vi "Process Repository.vi"(0 "Process In":refnum<class "Process.lvclass">, 5 "Action(ReadRepository)":T4(ring), 11 "Error In":errorcluster) -> (4 "Process Out":refnum<class "Process.lvclass">, 6 "ToProcessQueue":T2, 8 "ProcessAlreadyStarted":bool, 12 "ProcessViRef":refnum<vi>, 13 "ProcessSyncQueue":T3, 14 "FromProcessQueue":T1, 15 "Error Out":errorcluster)   [LabVIEW 2023, in "Process.lvclass"]
doc: "Governs the class object repository, in particular:\n- creates queues for new Process object, \n- allows impelement singleton pattern, \n- handles accesing to the process object queues,\n- menages liftime of queue storing process queues."
uses:
  Process.lvclass
  Interfaces/ICanCommunicate/ProcessSyncQueue.ctl
  Interfaces/ICanCommunicate/Message.ctl
  Interfaces/ICanCommunicate/ToProcessQueue.ctl
  Interfaces/ICanCommunicate/FromProcessQueue.ctl
  Interfaces/ICanCommunicate/Process Refs.ctl
  Process.lvclass/Process.ctl
  Process.vi
  Interfaces/ICanCommunicate/ICanCommunicate.lvclass
panel:
  # "Use this indicator for sending messages to the Process VI"
  # "These indicators are used by the process VIs"
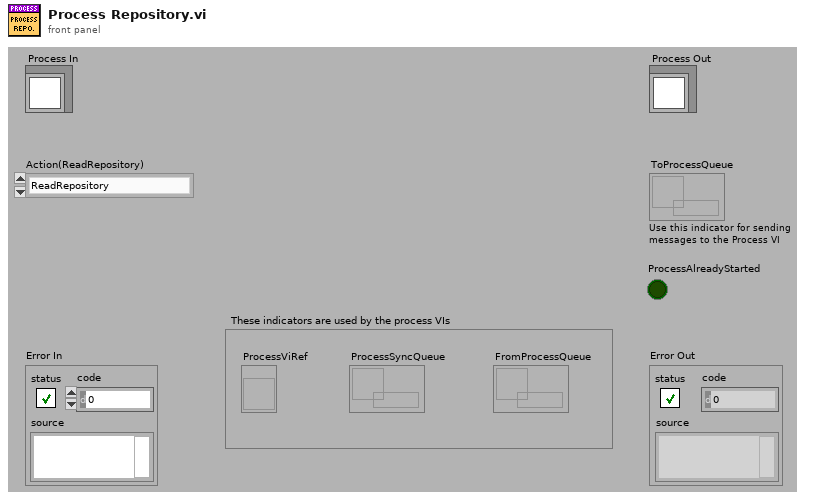
[diagram p1: front panel]
types:
  T1 = typedef "ICanCommunicate.lvclass/FromProcessQueue.ctl" = refnum<queue>
  T2 = typedef "ICanCommunicate.lvclass/ToProcessQueue.ctl" = refnum<queue>
  T3 = typedef "ICanCommunicate.lvclass/ProcessSyncQueue.ctl" = refnum<queue>
  T4 = enum16{"ReadRepository", "CreateNew", "CreateOrLookUpExisting", "ReadRepositoryAndDestroy"}
  T5 = typedef "ICanCommunicate.lvclass/Process Refs.ctl" = cluster{"ToProcessQueue":T2, "FromProcessQueue":T1, "ProcessSyncQueue":T3, "ProcessViRef":refnum<vi>}
  T6 = typedef "ICanCommunicate.lvclass/Message.ctl" = cluster{"Sender Name":string, "Recipent Name":string, "Command":string, "Data":variant, "Signature":string}
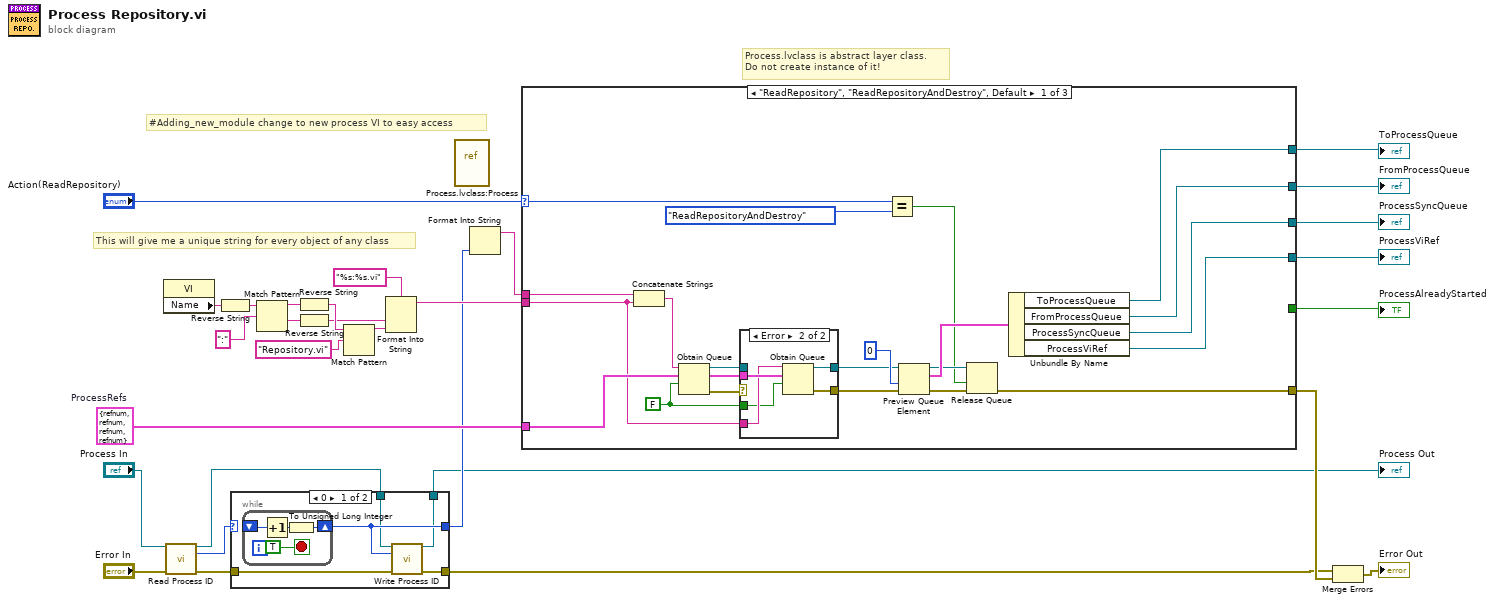
[diagram p0: block diagram]
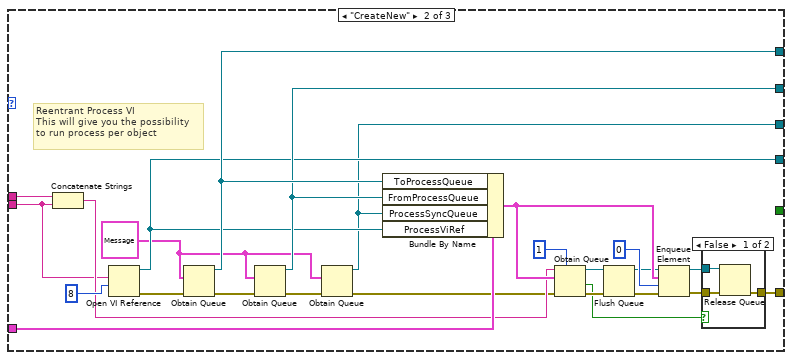
[diagram p4: hidden frame]
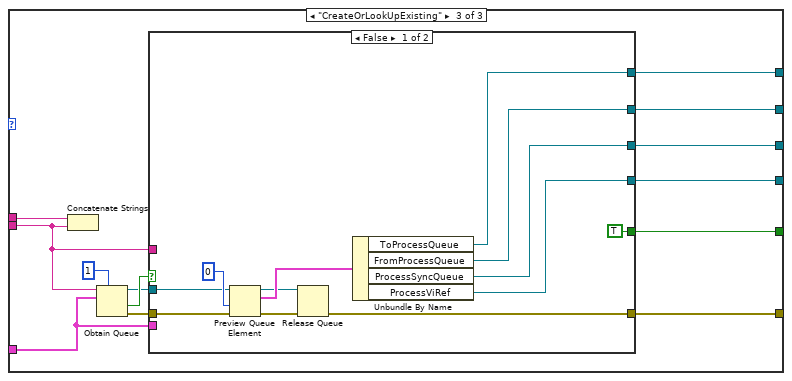
[diagram p6: hidden frame]
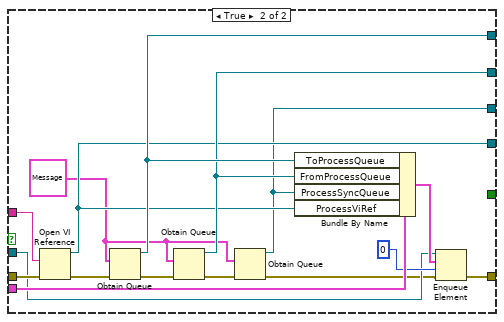
[diagram p7: hidden frame]
diagram:
  w24 = T5 {"ToProcessQueue"=refnum, "FromProcessQueue"=refnum, "ProcessSyncQueue"=refnum, "ProcessViRef"=refnum}  # ProcessRefs
  # "Process.lvclass is abstract layer class. \nDo not create instance of it!"
  # "#Adding_new_module change to new process VI to easy access"
  # "This will give me a unique string for every object of any class"
  n1 = property class="VI"() -> ("Name"=w13:string)  [unwired: 2 in, 2 out]
  n2 = call "Read Process ID.vi"("Process In"="Process In", "Error In"="Error In") -> ("Process Out"=w4:refnum<class "Process.lvclass">, "Process ID"=w2:u32, "Error Out"=w6:errorcluster)  [unwired: 11 in]
  n3 = Reverse String(1:w13) -> (0:w14:string)
  n4 = case shown="0" w2 {
    selector: w2 -> [_ w40]
    tunnel: [w34 w40] -> w7
    tunnel: w4 -> [w33 w41]
    tunnel: [w32 w41] -> w3
    tunnel: w6 -> [w31 w39]
    tunnel: [w30 w39] -> w8
    frame 0 {
      n5 = while {
        shift-right: [w35] -> w34
        shift-left: _ -> [w37]
        stop <- TRUE stop-if-true
        n6 = Increment(x=w37) -> (x+1=w36:u32)
        n7 = To Unsigned Long Integer(number=w36) -> (unsigned 32bit integer=w35:u32)
      }
      n8 = call "Write Process ID.vi"("Process In"=w33, "Process ID"=w34, "Error In"=w31) -> ("Process Out"=w32:refnum<class "Process.lvclass">, "Error Out"=w30:errorcluster)  [unwired: 11 in]
    }
    frame Default {
    }
  }
  "Process Out" <- w3
  n9 = Match Pattern(string=w14, regular expression=":") -> (before substring=w18:string, after substring=w15:string)  [unwired: 1 in, 2 out]
  n10 = Reverse String(1:w18) -> (0:w19:string)
  n11 = Reverse String(1:w15) -> (0:w17:string)
  n12 = Match Pattern(string=w19, regular expression="Repository.vi") -> (before substring=w21:string)  [unwired: 1 in, 3 out]
  n13 = Format Into String(format string="%s:%s.vi", w17, w21) -> (resulting string=w11:string)  [unwired: 2 in, 1 out]
  n14 = vi-ref "Process.lvclass:Process.vi"() -> ()  [unwired: 1 out]
  n15 = Format Into String(w7) -> (resulting string=w9:string)  [unwired: 3 in, 1 out]
  n16 = case shown="\"ReadRepository\", \"ReadRepositoryAndDestroy\", Default" "Action(ReadRepository)" {
    selector: "Action(ReadRepository)" -> [w43 _ _]
    tunnel: [w57 w78 w109] -> w28
    tunnel: [w59 w94 w111] -> w26
    tunnel: [w58 w93 w110] -> w27
    tunnel: [w60 w92 w108] -> w25
    tunnel: w24 -> [w52 w84 w104]
    tunnel: w9 -> [w50 w83 w100]
    tunnel: [w45 w72 w107] -> w22
    tunnel: w11 -> [w49 w81 w99]
    tunnel: [_ _ w102] -> w10
    frame "ReadRepository", "ReadRepositoryAndDestroy", Default {
      w51 = FALSE ("create if not found? (T)")
      n17 = Concatenate Strings(w50, w49) -> (w48:string)
      n18 = Obtain Queue(name (unnamed)=w48, element data type=w52, create if not found? (T)=w51) -> (queue out=w54:refnum<queue>, error out=w56:errorcluster)  [unwired: 2 in, 1 out]
      n19 = case shown="Error" w56 {
        selector: w56 -> [w64 _]
        tunnel: [w64 w66] -> w55
        tunnel: w54 -> [w63 _]
        tunnel: [w63 w67] -> w53
        tunnel: w52 -> [_ w69]
        tunnel: w49 -> [_ w68]
        tunnel: w51 -> [_ w65]
        frame No Error {
        }
        frame Error {
          n20 = Obtain Queue(name (unnamed)=w68, element data type=w69, create if not found? (T)=w65) -> (queue out=w67:refnum<queue>, error out=w66:errorcluster)  [unwired: 2 in, 1 out]
        }
      }
      n21 = Equal?(x=w43, y=T4."ReadRepositoryAndDestroy") -> (x = y?=w42:bool)
      n22 = Preview Queue Element(queue=w53, timeout in ms (-1)=0, error in (no error)=w55) -> (queue out=w47:refnum<queue>, element=w61:T5, error out=w46:errorcluster)  [unwired: 1 out]
      n23 = Release Queue(queue=w47, force destroy? (F)=w42, error in (no error)=w46) -> (error out=w45:errorcluster)  [unwired: 2 out]
      n24 = Unbundle By Name(w61) -> ("ToProcessQueue"=w59:T2, "FromProcessQueue"=w58:T1, "ProcessSyncQueue"=w57:T3, "ProcessViRef"=w60:refnum<vi>)
    }
    frame "CreateNew" {
      w70 = T6 {"Sender Name"="", "Recipent Name"="", "Command"="", "Data"=variant, "Signature"=""} ("Message")
      # "Reentrant Process VI\nThis will give you the possibility\nto run process per object"
      n25 = Concatenate Strings(w83, w81) -> (w82:string)
      n26 = Open VI Reference(vi path=w81, options=8 ("Reentrant Process VI\nThis will give you the possibility\nto run process per object")) -> (vi reference=w92:refnum<vi>, error out=w90:errorcluster)  [unwired: 4 in]
      n27 = Obtain Queue(element data type=w70, error in (no error)=w90) -> (queue out=w94:refnum<queue>, error out=w91:errorcluster)  [unwired: 3 in, 1 out]
      n28 = Obtain Queue(element data type=w70, error in (no error)=w91) -> (queue out=w93:refnum<queue>, error out=w80:errorcluster)  [unwired: 3 in, 1 out]
      n29 = Obtain Queue(element data type=w70, error in (no error)=w80) -> (queue out=w78:refnum<queue>, error out=w79:errorcluster)  [unwired: 3 in, 1 out]
      n30 = Bundle By Name(cluster=w84, "ToProcessQueue"=w94, "FromProcessQueue"=w93, "ProcessSyncQueue"=w78, "ProcessViRef"=w92) -> (w87:T5)
      n31 = Obtain Queue(max queue size (-1, unlimited)=1, name (unnamed)=w82, element data type=w87, error in (no error)=w79) -> (queue out=w88:refnum<queue>, created new?=w71:bool, error out=w76:errorcluster)  [unwired: 1 in]
      n32 = Flush Queue(queue=w88, error in (no error)=w76) -> (queue out=w77:refnum<queue>, error out=w75:errorcluster)  [unwired: 1 out]
      n33 = Enqueue Element(queue=w77, element=w87, timeout in ms (-1)=0, error in (no error)=w75) -> (queue out=w74:refnum<queue>, error out=w73:errorcluster)  [unwired: 1 out]
      n34 = case shown="False" w71 {
        tunnel: w73 -> [w97 w98]
        tunnel: w74 -> [w96 _]
        tunnel: [w95 w98] -> w72
        frame False {
          n35 = Release Queue(queue=w96, error in (no error)=w97) -> (error out=w95:errorcluster)  [unwired: 1 in, 2 out]
        }
        frame True {
        }
      }
    }
    frame "CreateOrLookUpExisting" {
      n36 = Concatenate Strings(w100, w99) -> ()  [unwired: 1 out]
      n37 = Obtain Queue(max queue size (-1, unlimited)=1, name (unnamed)=w99, element data type=w104) -> (queue out=w105:refnum<queue>, created new?=w106:bool, error out=w103:errorcluster)  [unwired: 2 in]
      n38 = case shown="False" w106 {
        tunnel: [w123 w139] -> w111
        tunnel: [w122 w138] -> w110
        tunnel: [w121 w125] -> w109
        tunnel: [w120 w137] -> w108
        tunnel: [w112 w136] -> w107
        tunnel: w104 -> [_ w135]
        tunnel: w103 -> [w117 w130]
        tunnel: w99 -> [_ w129]
        tunnel: w105 -> [w118 w128]
        tunnel: [TRUE _] -> w102
        frame False {
          n39 = Preview Queue Element(queue=w118, timeout in ms (-1)=0, error in (no error)=w117) -> (queue out=w114:refnum<queue>, element=w116:T5, error out=w113:errorcluster)  [unwired: 1 out]
          n40 = Release Queue(queue=w114, error in (no error)=w113) -> (error out=w112:errorcluster)  [unwired: 1 in, 2 out]
          n41 = Unbundle By Name(w116) -> ("ToProcessQueue"=w123:T2, "FromProcessQueue"=w122:T1, "ProcessSyncQueue"=w121:T3, "ProcessViRef"=w120:refnum<vi>)
        }
        frame True {
          w124 = T6 {"Sender Name"="", "Recipent Name"="", "Command"="", "Data"=variant, "Signature"=""} ("Message")
          n42 = Open VI Reference(vi path=w129, error in (no error)=w130) -> (vi reference=w137:refnum<vi>, error out=w133:errorcluster)  [unwired: 4 in]
          n43 = Obtain Queue(element data type=w124, error in (no error)=w133) -> (queue out=w139:refnum<queue>, error out=w134:errorcluster)  [unwired: 3 in, 1 out]
          n44 = Obtain Queue(element data type=w124, error in (no error)=w134) -> (queue out=w138:refnum<queue>, error out=w127:errorcluster)  [unwired: 3 in, 1 out]
          n45 = Obtain Queue(element data type=w124, error in (no error)=w127) -> (queue out=w125:refnum<queue>, error out=w126:errorcluster)  [unwired: 3 in, 1 out]
          n46 = Bundle By Name(cluster=w135, "ToProcessQueue"=w139, "FromProcessQueue"=w138, "ProcessSyncQueue"=w125, "ProcessViRef"=w137) -> (w132:T5)
          n47 = Enqueue Element(queue=w128, element=w132, timeout in ms (-1)=0, error in (no error)=w126) -> (error out=w136:errorcluster)  [unwired: 2 out]
        }
      }
    }
  }
  "ProcessSyncQueue" <- w28
  "ToProcessQueue" <- w26
  "FromProcessQueue" <- w27
  "ProcessViRef" <- w25
  "ProcessAlreadyStarted" <- w10
  n48 = Merge Errors(w8, w22) -> (→"Error Out":errorcluster)
